vi "sensor cmd bootloader version.vi"(10 "dest_version":u32, 11 "device_handle":u32) -> (1 "function return":i32, 2 "dest_version out":u32, 3 "device_handle out":u32)   [LabVIEW 2019, in "apdm.lvlib"]
doc: "APDM_EXPORT int apdm_sensor_cmd_bootloader_version(apdm_device_handle_t device_handle, uint32_t *dest_version);"
uses:
  apdm.lvlib
  Lee Lab/CP FES Walking 2018/Code/Working/LabVIEW/apdm.dll
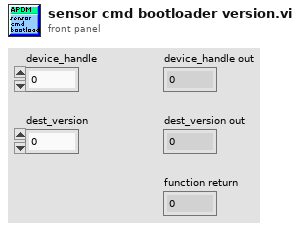
[diagram p1: front panel]
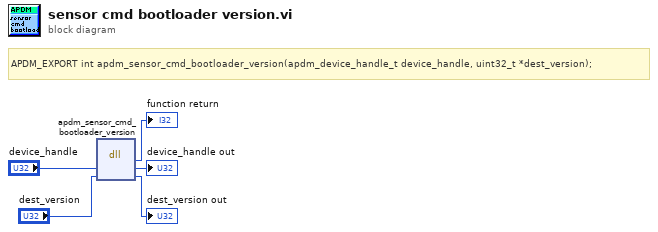
[diagram p0: block diagram]
diagram:
  # "APDM_EXPORT int apdm_sensor_cmd_bootloader_version(apdm_device_handle_t device_handle, uint32_t *dest_version);"
  n1 = dll-call lib="C:/Users/jfalesi/Dropbox/Lee Lab/CP FES Walking 2018/Code/Working/LabVIEW/apdm.*" fn="apdm_sensor_cmd_bootloader_version"("device_handle"="device_handle", "dest_version"="dest_version") -> (→"function return":i32, "device_handle"=→"device_handle out":u32, "dest_version"=→"dest_version out":u32)  [unwired: 3 in, 2 out]
